vi "Write HART resource name.vi"(8 "error in (no error)":errorcluster, 10 "HART resource name":refnum<visa-resource-name>="HART", 11 "HART in":refnum<class "HART.lvclass">) -> (0 "error out":errorcluster, 3 "HART out":refnum<class "HART.lvclass">)   [LabVIEW 2016, in "HART.lvclass"]
uses:
  HART.lvclass
  HART.lvclass/HART.ctl
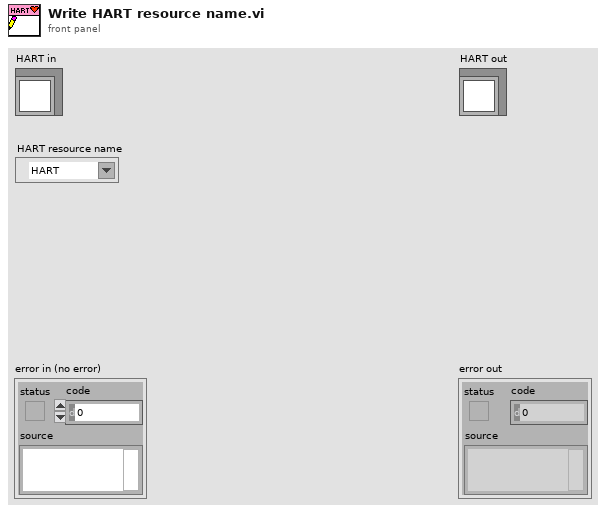
[diagram p1: front panel]
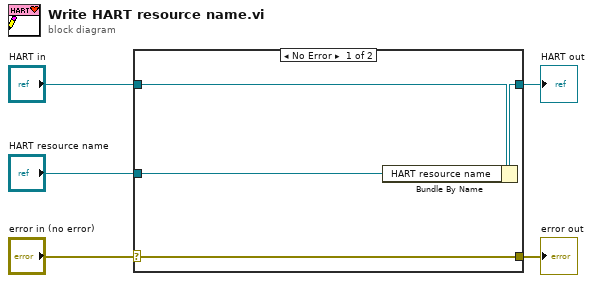
[diagram p0: block diagram]
diagram:
  n1 = case shown="No Error" "error in (no error)" {
    selector: "error in (no error)" -> [w9 w10]
    tunnel: [w9 w10] -> w4
    tunnel: [w7 w11] -> w2
    tunnel: "HART in" -> [w8 w11]
    tunnel: "HART resource name" -> [w6 _]
    frame No Error {
      n2 = Bundle By Name(cluster=w8, "HART resource name"=w6) -> (w7:refnum<class "HART.lvclass">)
    }
    frame Error {
    }
  }
  "error out" <- w4
  "HART out" <- w2
